vi "MGI progress bar example.vi"   [LabVIEW 2013]
uses:
  <userlib>/_MGI/User Interface/Progress Bar/Progress Bar.lvclass
  <userlib>/_MGI/User Interface/Progress Bar/Progress Bar Settings/Progress Bar Settings.lvclass
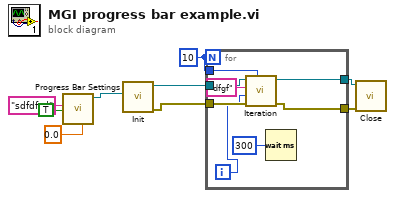
[diagram p0: block diagram]
diagram:
  w9 = 10
  n1 = call <userlib>:"Progress Bar Settings.vi"("Seconds Before Showing (1)"=0.0, "Window Title (Progress)"="sdfdfsd", "Show Abort (f)"=TRUE) -> ("MGI_Progress Bar Settings"=w4:refnum<class "Progress Bar Settings.lvclass">)  [unwired: 8 in]
  n2 = call <userlib>:"Init.vi"("Settings"=w4) -> ("error out"=w7:errorcluster, "Progress Bar"=w8:refnum<data-value>)  [unwired: 9 in]
  n3 = for {
    N: w9 -> [_]
    tunnel: w9 -> [w16]
    tunnel: w8 -> [w15]
    tunnel: w7 -> [w14]
    tunnel: [w13] -> w6
    tunnel: [w12] -> w5
    i -> [w10]
    n4 = call <userlib>:"Iteration.vi"("Total Iterations"=w16, "error in (no error)"=w14, "Current Iteration"=w10, "Message"="dfgf", "Progress Bar"=w15) -> ("error out"=w12:errorcluster, "Progress Bar"=w13:refnum<data-value>)  [unwired: 4 in, 1 out]
    n5 = Wait (ms)(milliseconds to wait=u32 300) -> ()  [unwired: 1 out]
  }
  n6 = call <userlib>:"Close.vi"("error in (no error)"=w5, "Progress Bar"=w6) -> ()  [unwired: 9 in, 1 out]
